vi "ADC_READ VHLTHx VLLTHx muy simple.vi"(0 "ftHandle_out 2":u32, 1 "Sumador":u8, 5 "error out 2":errorcluster, 8 "Espera acceso FT":u32) -> (14 "ftHandle_out":u32, 15 "HLTHx":dbl, 16 "LLTHx":dbl, 19 "error out":errorcluster)   [LabVIEW 2019]
uses:
  ASIC_Valores dac_mux_ena.ctl
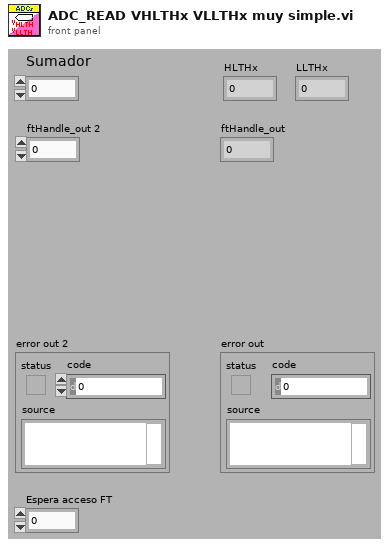
[diagram p1: front panel]
types:
  T1 = typedef "ASIC_Valores dac_mux_ena.ctl" = enum16{"---NULL 0--", "HLTH0 (ADD A)", "HLTH1 (ADD B)", "HLTH2 (ADD C)", "LLTH0 (ADD A)", "LLTH1 (ADD B)", "LLTH2 (ADD C)", "---NULL 1--"}
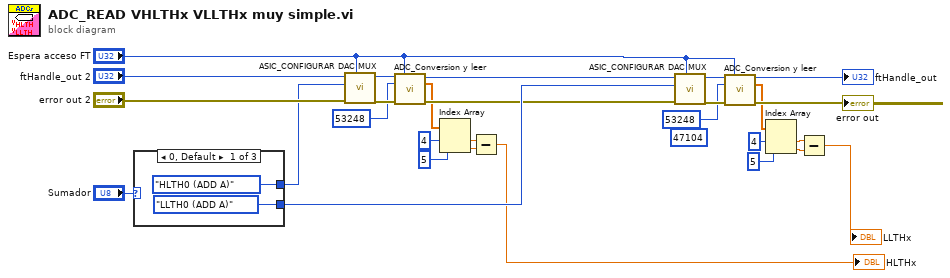
[diagram p0: block diagram]
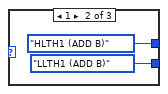
[diagram p2: hidden frame]
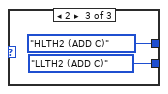
[diagram p3: hidden frame]
diagram:
  (unwired) u16 47104
  n1 = case shown="0, Default" "Sumador" {
    tunnel: [ASIC_Valores_dac_mux_ena."HLTH0 (ADD A)" ("dac mux(0..7)") ASIC_Valores_dac_mux_ena."HLTH1 (ADD B)" ("dac mux(0..7)") ASIC_Valores_dac_mux_ena."HLTH2 (ADD C)" ("dac mux(0..7)")] -> w25
    tunnel: [ASIC_Valores_dac_mux_ena."LLTH0 (ADD A)" ("dac mux(0..7)") ASIC_Valores_dac_mux_ena."LLTH1 (ADD B)" ("dac mux(0..7)") ASIC_Valores_dac_mux_ena."LLTH2 (ADD C)" ("dac mux(0..7)")] -> w22
    frame 0, Default {
    }
    frame 1 {
    }
    frame 2 {
    }
  }
  n2 = call "ASIC_CONFIGURAR DAC MUX.vi"("Espera acceso USB"="Espera acceso FT", "error in"="error out 2", "dac mux(0..7)"=w25, "ftHandle_in"="ftHandle_out 2") -> ("error out"=w11:errorcluster, "ftHandle_out"=w10:u32)  [unwired: 5 in, 1 out]
  n3 = call "ADC_Conversion y leer.vi"("ftHandle_in 2"=w10, "Espera acceso USB"="Espera acceso FT", "Registro Conversion (0xD000)"=u16 53248, "error in 2"=w11) -> ("ftHandle_out"=w23:u32, "Datos Canal (V)"=w12:dbl[], "error out"=w21:errorcluster)  [unwired: 6 in, 3 out]
  n4 = Index Array(array=w12, index #1=4 ("index"), index #2=5 ("index")) -> (element #1=w15:dbl, element #2=w16:dbl)
  n5 = Subtract(x=w15, y=w16) -> (x-y=→"HLTHx":dbl)
  n6 = call "ASIC_CONFIGURAR DAC MUX.vi"("Espera acceso USB"="Espera acceso FT", "error in"=w21, "dac mux(0..7)"=w22, "ftHandle_in"=w23) -> ("error out"=w4:errorcluster, "ftHandle_out"=w3:u32)  [unwired: 5 in, 1 out]
  n7 = call "ADC_Conversion y leer.vi"("ftHandle_in 2"=w3, "Espera acceso USB"="Espera acceso FT", "Registro Conversion (0xD000)"=u16 53248, "error in 2"=w4) -> ("ftHandle_out"=→"ftHandle_out":u32, "Datos Canal (V)"=w5:dbl[], "error out"=→"error out":errorcluster)  [unwired: 6 in, 3 out]
  n8 = Index Array(array=w5, index #1=4 ("index"), index #2=5 ("index")) -> (element #1=w7:dbl, element #2=w8:dbl)
  n9 = Subtract(x=w7, y=w8) -> (x-y=→"LLTHx":dbl)
